vi "Close MeasurementLink Session.vi"(8 "error in":errorcluster, 9 "initialize and close session behavior":T1, 10 "session in":variant, 11 "session factory in":refnum<class "Session Factory.lvclass">) -> (0 "error out":errorcluster)   [LabVIEW 2021, in "NI Session Management niDigital.lvlib" / "Session Factory.lvclass"]
uses:
  Session Factory.lvclass
  Instrument/ISession Factory/Initialize and Close Session Behavior.ctl
  Instrument/ISession Factory/ISession Factory.lvclass
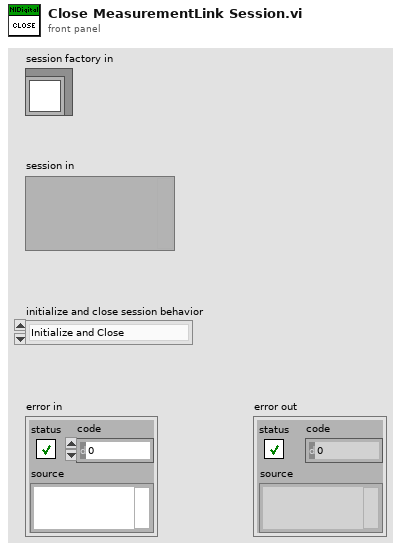
[diagram p1: front panel]
types:
  T1 = typedef "NI Session Management Instrument.lvlib/ISession Factory.lvclass/Initialize and Close Session Behavior.ctl" = enum16{"Initialize and Close", "Attach and Detach", "Initialize and Detach", "Attach and Close"}
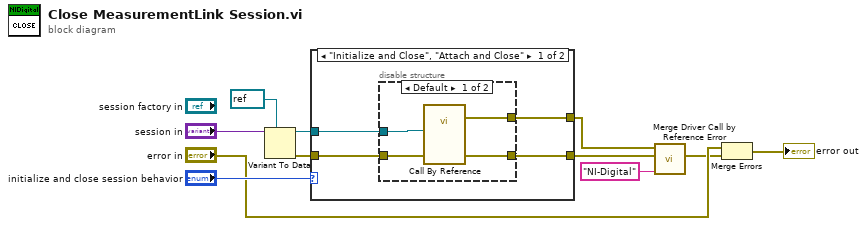
[diagram p0: block diagram]
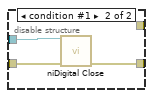
[diagram p2: hidden frame]
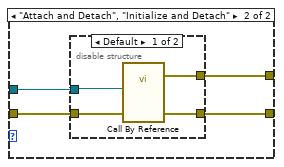
[diagram p3: hidden frame]
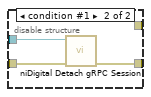
[diagram p4: hidden frame]
diagram:
  n1 = Variant To Data(type=refnum<k15> refnum ("instrument handle"), Variant="session in") -> (data=w8:refnum<k15>, error out=w9:errorcluster)  [unwired: 1 in]
  n2 = case shown="\"Initialize and Close\", \"Attach and Close\"" "initialize and close session behavior" {
    tunnel: w9 -> [w15 w26]
    tunnel: w8 -> [w14 w24]
    tunnel: [w13 w25] -> w2
    tunnel: [w12 w23] -> w1
    frame "Initialize and Close", "Attach and Close" {
      n3 = disable-structure shown="Default" {
        disable-tunnel: w15 -> [w19 w22]
        disable-tunnel: w14 -> [w18 w21]
        disable-tunnel: [w17 w20] -> w13
        disable-tunnel: [w16 _] -> w12
        frame condition #0 (active) {
          n4 = call-by-ref "?"("instrument handle"=w18, "error in"=w19) -> (error out=w16:errorcluster, 15:"error out"=w17:errorcluster)  [unwired: 15 in, 1 out]
        }
        frame condition #1 {
          n5 = call <instrlib>:"niDigital Close.vi"("instrument handle"=w21, "error in"=w22) -> ("error out"=w20:errorcluster)  [unwired: 13 in]
        }
      }
    }
    frame "Attach and Detach", "Initialize and Detach" {
      n6 = disable-structure shown="Default" {
        disable-tunnel: w26 -> [w30 w33]
        disable-tunnel: [w29 w32] -> w25
        disable-tunnel: w24 -> [w28 w31]
        disable-tunnel: [w27 _] -> w23
        frame condition #0 (active) {
          n7 = call-by-ref "?"("instrument handle"=w28, "error in"=w30) -> (error out=w27:errorcluster, 15:"error out"=w29:errorcluster)  [unwired: 15 in, 1 out]
        }
        frame condition #1 {
          n8 = call <instrlib>:"niDigital Detach gRPC Session.vi"("instrument handle"=w31, "error in"=w33) -> ("error out"=w32:errorcluster)  [unwired: 13 in]
        }
      }
    }
  }
  n9 = call "Merge Driver Call by Reference Error.vi"("driver name"="NI-Digital", "called vi error"=w2, "call by ref error"=w1) -> ("error out"=w3:errorcluster)  [unwired: 8 in]
  n10 = Merge Errors("error in", w3) -> (→"error out":errorcluster)
